vi "Init.vi"(8 "No Error":errorcluster) -> (0 "error out":errorcluster)   [LabVIEW 2024, in "SDL3.lvlib" / "TTF.lvlib"]
doc: "<B>Summary</B>\nInitialize SDL_ttf.\n\n<B>Remarks</B>\nYou must successfully call this function before it is safe to call any other function in this library.\n\nIt is safe to call this more than once, and each successful <B>TTF_Init()</B> call should be paired with a matching <B>TTF_Quit()</B> call."
uses:
  TTF.lvlib
  Error/Error.lvlib
  Lib/Win32/SDL3_ttf/SDL3_ttf.dll
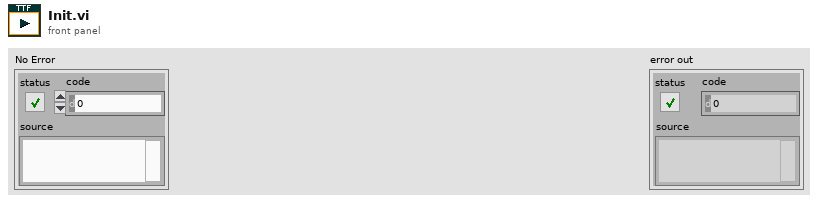
[diagram p1: front panel]
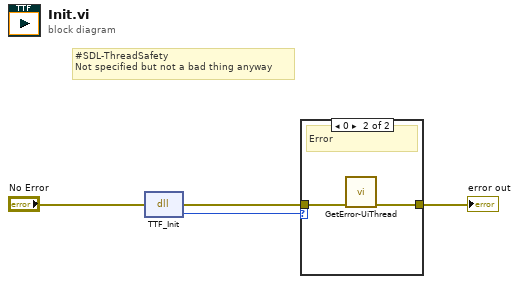
[diagram p0: block diagram]
diagram:
  # "#SDL-ThreadSafety\nNot specified but not a bad thing anyway"
  n1 = dll-call lib="C:/Users/Thomas/Documents/Projects/LV-SDL3/Lib/Win32/SDL3_ttf/SDL3_ttf.dll" fn="TTF_Init"(error in="No Error") -> (error out=w1:errorcluster, "return type"=w2:i32)  [unwired: 2 in, 1 out]
  n2 = case shown="0" w2 {
    tunnel: w1 -> [w5 w7]
    tunnel: [w5 w6] -> w3
    frame Default {
      # "Ok"
    }
    frame 0 {
      # "Error"
      n3 = call "GetError-UiThread.vi"("No Error"=w7) -> ("error out"=w6:errorcluster)  [unwired: 10 in]
    }
  }
  "error out" <- w3
